vi "LabVIEW Dependencies Path.vi"(11 "error in":errorcluster) -> (4 "vilib path":path, 6 "arrange bd path":path, 8 "arrange fp path":path, 15 "error out":errorcluster)   [LabVIEW 2021, in "Path Functions.lvlib"]
uses:
  Path Functions.lvlib
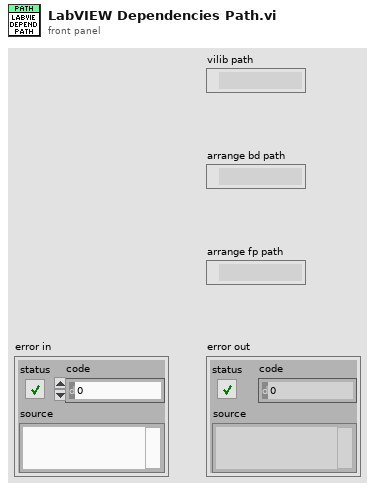
[diagram p1: front panel]
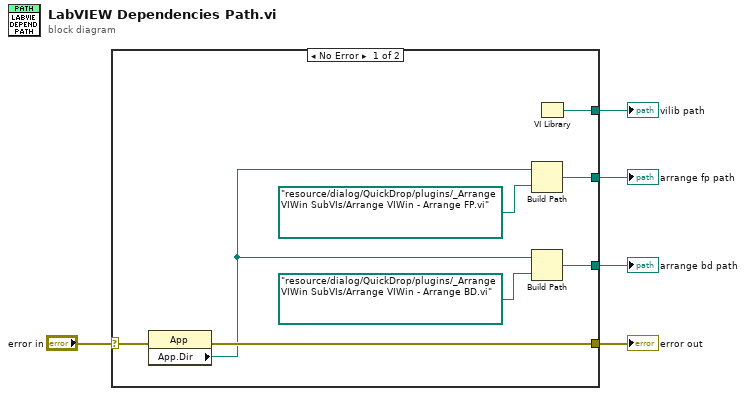
[diagram p0: block diagram]
diagram:
  n1 = case shown="No Error" "error in" {
    selector: "error in" -> [w11 w14]
    tunnel: [w13 _] -> w5
    tunnel: [w12 _] -> w4
    tunnel: [w10 w14] -> w3
    tunnel: [w6 _] -> w1
    frame No Error {
      n2 = property class="App"(error in=w11) -> (error out=w10:errorcluster, "App.Dir"=w9:path)  [unwired: 1 in, 1 out]
      n3 = Build Path(base path=w9, name or relative path=path "resource/dialog/QuickDrop/plugins/_Arrange VIWin SubVIs/Arrange VIWin - Arrange FP.vi") -> (appended path=w13:path)
      n4 = Build Path(base path=w9, name or relative path=path "resource/dialog/QuickDrop/plugins/_Arrange VIWin SubVIs/Arrange VIWin - Arrange BD.vi") -> (appended path=w12:path)
      n5 = VI Library() -> (path=w6:path)
    }
    frame Error {
    }
  }
  "vilib path" <- w1
  "arrange fp path" <- w5
  "arrange bd path" <- w4
  "error out" <- w3
